vi "TXT_Read.vi"(4 "error in (no error)":errorcluster, 5 "Configuration for text file":T1, 7 "Path of ABF file":path=path "D:/bme/abffile/demo3.abf") -> (0 "error out":errorcluster, 1 "Cell ID":string, 2 "File Paramters":T2, 3 "Whole Trace":sgl[][](array[numeric]))   [LabVIEW 2017]
uses:
  <vilib>/Utility/file.llb/Read Delimited Spreadsheet (DBL).vi
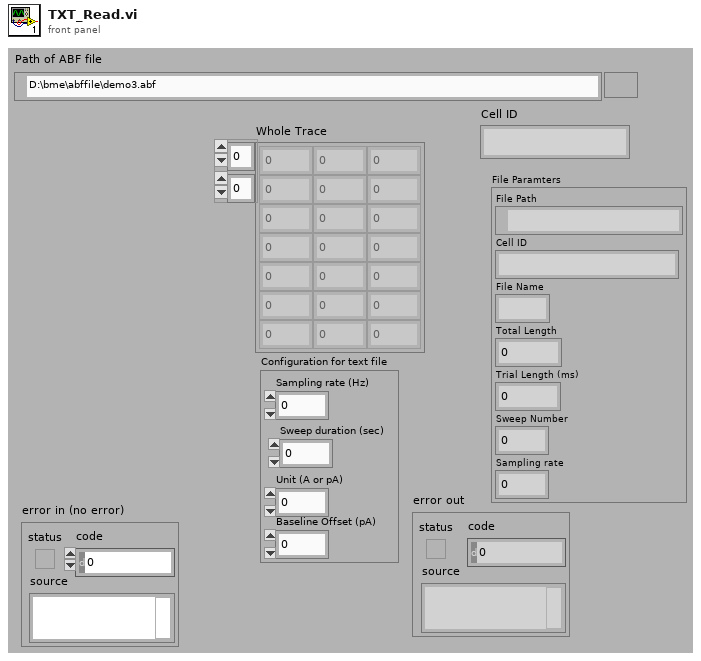
[diagram p1: front panel]
types:
  T1 = cluster{"Sampling rate (Hz)":dbl, "Sweep duration (sec)":dbl, "Unit (A or pA)":u16, "Baseline Offset (pA)":dbl}
  T2 = cluster{"File Path":path, "Cell ID":string, "File Name":string, "Total Length":i32, "Trial Length (ms)":dbl, "Sweep Number":dbl, "Sampling rate":dbl}
  T3 = cluster{"stripped path":path, "name":string, "name":string, dbl, dbl, i32, "Sampling rate (Hz)":dbl}
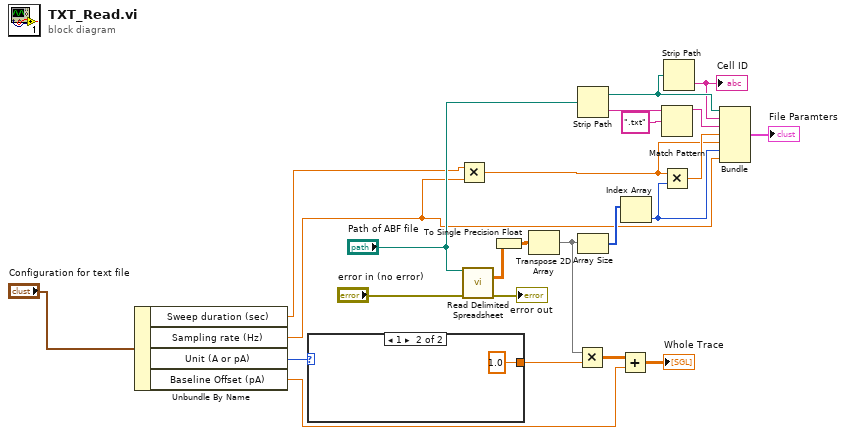
[diagram p0: block diagram]
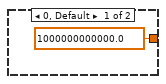
[diagram p2: hidden frame]
diagram:
  n1 = Unbundle By Name("Configuration for text file") -> ("Sweep duration (sec)"=w3:dbl, "Sampling rate (Hz)"=w2:dbl, "Unit (A or pA)"=w8:u16, "Baseline Offset (pA)"=w7:dbl)
  n2 = case shown="1" w8 {
    tunnel: [1000000000000.0 1.0] -> w11
    frame 0, Default {
    }
    frame 1 {
    }
  }
  n3 = Multiply(x=w3, y=w2) -> (x*y=w1:dbl)
  n4 = call-poly <vilib>:"Read Delimited Spreadsheet.vi"("file path (dialog if empty)"="Path of ABF file", "error in (no error)"="error in (no error)") -> ("all rows"=w6:dbl[][], "error out"=→"error out":errorcluster)  [unwired: 8 in, 4 out]
  n5 = To Single Precision Float(number=w6) -> (single precision float=w5:sgl[][])
  n6 = Transpose 2D Array(2D array=w5) -> (transposed array=w12:sgl[][])
  n7 = Multiply(x=w12, y=w11) -> (x*y=w10:dbl[][])
  n8 = Strip Path(path="Path of ABF file") -> (stripped path=w24:path, name=w23:string)
  n9 = Array Size(array=w12) -> (size(s)=w15:i32[])
  n10 = Add(x=w10, y=w7) -> (x+y=→"Whole Trace":dbl[][])
  n11 = Index Array(array=w15) -> (element=w14:i32)  [unwired: 1 in]
  n12 = Match Pattern(string=w23, regular expression=".txt" ("정규식")) -> (before substring=w22:string)  [unwired: 1 in, 3 out]
  n13 = Multiply(x=w1, y=w14) -> (x*y=w13:dbl)
  n14 = Strip Path(path=w24) -> (name=w21:string)  [unwired: 1 out]
  "Cell ID" <- w21
  n15 = Bundle("stripped path"=w24, "name"=w21, "name"=w22, w13, w1, w14, "Sampling rate (Hz)"=w2) -> (→"File Paramters":T3)  [unwired: 1 in]
